vi "Intialize Caraya.vi"   [LabVIEW 2020]
uses:
  <vilib>/addons/_JKI Toolkits/Caraya/classes/Assert/Assert True.vi
  <vilib>/addons/_JKI Toolkits/Caraya/classes/Test/Test.lvclass
  <vilib>/addons/_JKI Toolkits/Caraya/classes/Assert/Assert.lvclass
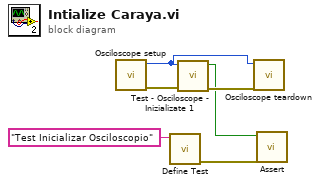
[diagram p0: block diagram]
diagram:
  n1 = call "Osciloscope setup.vi"() -> ("error out"=w4:errorcluster, "Module ID"=w1:i32)  [unwired: 10 in]
  n2 = call <vilib>:"Define Test.vi"("Label (VI Title)"="Test Inicializar Osciloscopio") -> ("error out"=w6:errorcluster)  [unwired: 10 in]
  n3 = call "Test - Osciloscope - Inizializate 1.vi"("error in (no error)"=w4, "Module ID"=w1) -> ("error out"=w3:errorcluster, "Pass"=w2:bool)  [unwired: 8 in]
  n4 = call "Osciloscope teardown.vi"("error in"=w3, "Module ID"=w1) -> ()  [unwired: 9 in, 1 out]
  n5 = call-poly <vilib>:"Assert.vi"("error in (no error)"=w6, "True?"=w2) -> ()  [unwired: 9 in, 1 out]
